vi "Controller Extract FOFB Variables.vi"(8 "error in (no error)":errorcluster, 11 "FOFB Configuration":T1) -> (0 "error out":errorcluster, 3 "FOFB Variables":T10)   [LabVIEW 2011, in "Controller VIs.lvlib"]
uses:
  Controller VIs.lvlib
  Types Definitions/Type FOFB Variables.ctl
  Types Definitions/Type FOFB Configuration.ctl
  Types Definitions/Type FOFB Parameters.ctl
  Types Definitions/Type Network Configuration.ctl
  Types Definitions/Type FA Configuration.ctl
  Types Definitions/Type Response Matrix Measurement Configuration.ctl
  Types Definitions/Type Correction Algorithm Configuration.ctl
  Types Definitions/Type Acquisition Network Configuration.ctl
  Types Definitions/Type Actuation Network Configuration.ctl
  Types Definitions/Type PID Parameters.ctl
  Type Definitions.lvlib
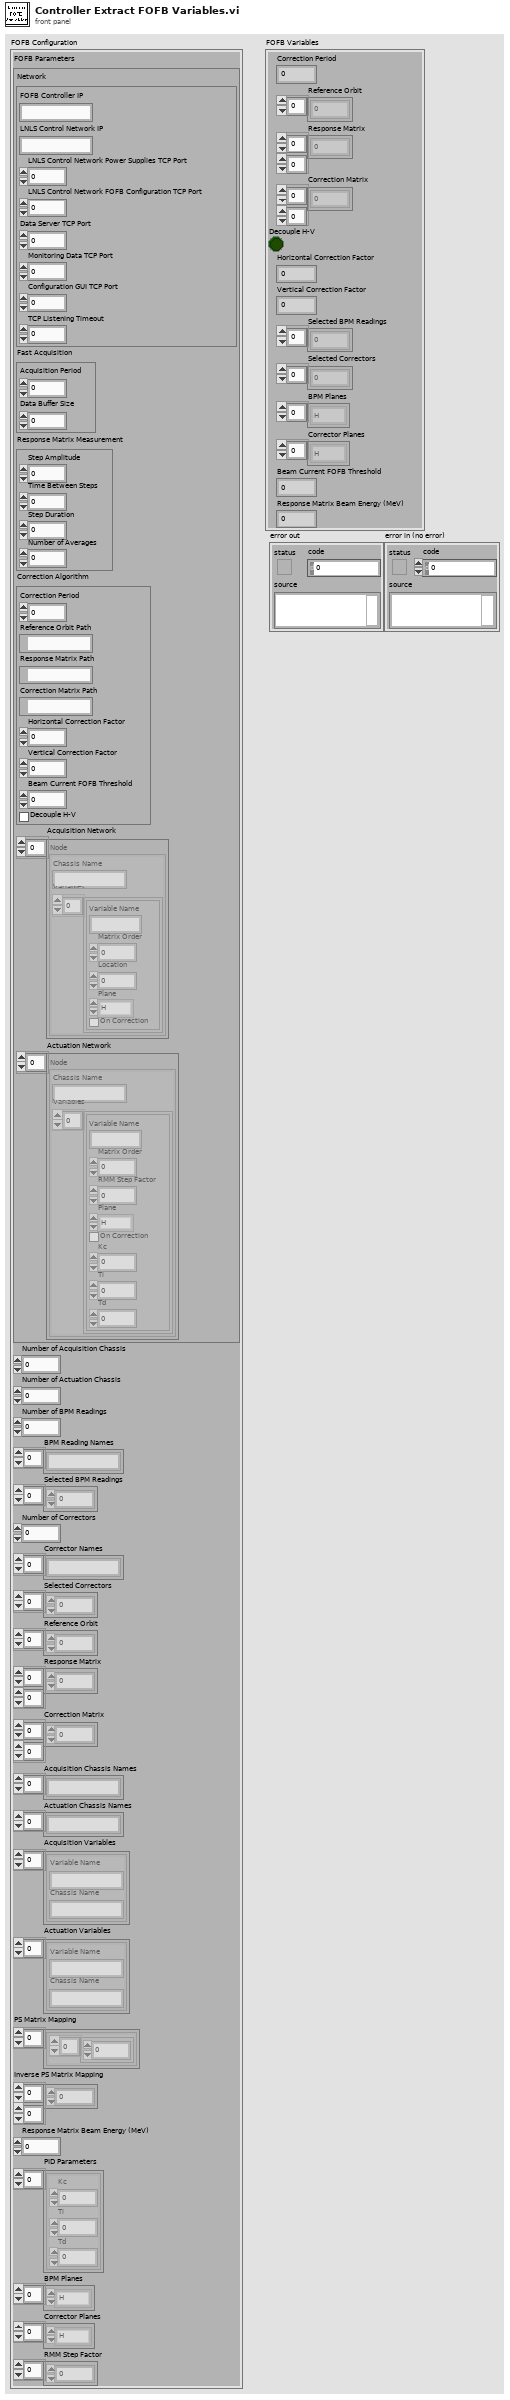
[diagram p1: front panel]
types:
  T1 = typedef "Type Definitions.lvlib/Type FOFB Configuration.ctl" = cluster{"FOFB Parameters":T2, "Number of Acquisition Chassis":i32, "Number of Actuation Chassis":i32, "Number of BPM Readings":i32, "BPM Reading Names":string[], "Selected BPM Readings":u32[], "Number of Correctors":i32, "Corrector Names":string[], "Selected Correctors":u32[], "Reference Orbit":dbl[], "Response Matrix":dbl[][], "Correction Matrix":dbl[][], "Acquisition Chassis Names":string[], "Actuation Chassis Names":string[], "Acquisition Variables":cluster{"Variable Name":string, "Chassis Name":string}[], "Actuation Variables":cluster{"Variable Name":string, "Chassis Name":string}[], "PS Matrix Mapping":cluster{u32[]}[], "Inverse PS Matrix Mapping":u32[][], "Response Matrix Beam Energy (MeV)":dbl, "PID Parameters":T9[], "BPM Planes":enum8{"H", "V"}[], "Corrector Planes":enum8{"H", "V"}[], "RMM Step Factor":dbl[]}
  T2 = typedef "Type Definitions.lvlib/Type FOFB Parameters.ctl" = cluster{"Network":T3, "Fast Acquisition":T4, "Response Matrix Measurement":T5, "Correction Algorithm":T6, "Acquisition Network":T7, "Actuation Network":T8}
  T3 = typedef "Type Definitions.lvlib/Type Network Configuration.ctl" = cluster{"FOFB Controller IP":string, "LNLS Control Network IP":string, "LNLS Control Network Power Supplies TCP Port":u16, "LNLS Control Network FOFB Configuration TCP Port":u16, "Data Server TCP Port":u16, "Monitoring Data TCP Port":u16, "Configuration GUI TCP Port":u16, "TCP Listening Timeout":i32}
  T4 = typedef "Type Definitions.lvlib/Type FA Configuration.ctl" = cluster{"Acquisition Period":u32, "Data Buffer Size":u32}
  T5 = typedef "Type Definitions.lvlib/Type Response Matrix Measurement Configuration.ctl" = cluster{"Step Amplitude":dbl, "Time Between Steps":u32, "Step Duration":u32, "Number of Averages":u32}
  T6 = typedef "Type Definitions.lvlib/Type Correction Algorithm Configuration.ctl" = cluster{"Correction Period":u32, "Reference Orbit Path":path, "Response Matrix Path":path, "Correction Matrix Path":path, "Horizontal Correction Factor":dbl, "Vertical Correction Factor":dbl, "Beam Current FOFB Threshold":dbl, "Decouple H-V":bool}
  T7 = typedef "Type Definitions.lvlib/Type Acquisition Network Configuration.ctl" = cluster{"Chassis Name":string, "Variables":cluster{"Variable Name":string, "Matrix Order":u32, "Location":dbl, "Plane":enum8{"H", "V"}, "On Correction":bool}[]}[]
  T8 = typedef "Type Definitions.lvlib/Type Actuation Network Configuration.ctl" = cluster{"Chassis Name":string, "Variables":cluster{"Variable Name":string, "Matrix Order":u32, "RMM Step Factor":dbl, "Plane":enum8{"H", "V"}, "On Correction":bool, "Kc":dbl, "Ti":dbl, "Td":dbl}[]}[]
  T9 = typedef "Type Definitions.lvlib/Type PID Parameters.ctl" = cluster{"Kc":fxp<+/-,16,8>, "Ti":fxp<+/-,16,8>, "Td":fxp<+/-,16,8>}
  T10 = typedef "Type Definitions.lvlib/Type FOFB Variables.ctl" = cluster{"Correction Period":u32, "Reference Orbit":dbl[], "Response Matrix":dbl[][], "Correction Matrix":dbl[][], "Decouple H-V":bool, "Horizontal Correction Factor":dbl, "Vertical Correction Factor":dbl, "Selected BPM Readings":u32[], "Selected Correctors":u32[], "BPM Planes":enum8{"H", "V"}[], "Corrector Planes":enum8{"H", "V"}[], "Beam Current FOFB Threshold":dbl, "Response Matrix Beam Energy (MeV)":dbl}
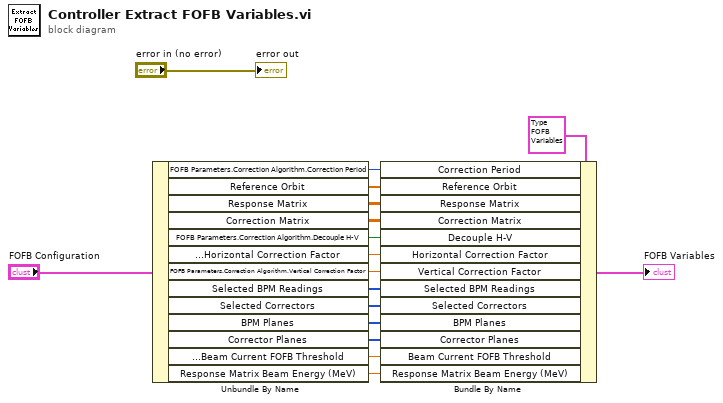
[diagram p0: block diagram]
diagram:
  n1 = Unbundle By Name("FOFB Configuration") -> ("FOFB Parameters.Correction Algorithm.Correction Period"=w15:u32, "Reference Orbit"=w14:dbl[], "Response Matrix"=w13:dbl[][], "Correction Matrix"=w12:dbl[][], "FOFB Parameters.Correction Algorithm.Decouple H-V"=w11:bool, "FOFB Parameters.Correction Algorithm.Horizontal Correction Factor"=w10:dbl, "FOFB Parameters.Correction Algorithm.Vertical Correction Factor"=w9:dbl, "Selected BPM Readings"=w8:u32[], "Selected Correctors"=w7:u32[], "BPM Planes"=w6:enum8{"H", "V"}[], "Corrector Planes"=w5:enum8{"H", "V"}[], "FOFB Parameters.Correction Algorithm.Beam Current FOFB Threshold"=w4:dbl, "Response Matrix Beam Energy (MeV)"=w3:dbl)
  n2 = Bundle By Name(cluster=T10 {"Correction Period"=0, "Reference Orbit"=[], "Response Matrix"=[], "Correction Matrix"=[], "Decouple H-V"=FALSE, "Horizontal Correction Factor"=0.0, "Vertical Correction Factor"=0.0, "Selected BPM Readings"=[], "Selected Correctors"=[], "BPM Planes"=[], "Corrector Planes"=[], "Beam Current FOFB Threshold"=0.0, "Response Matrix Beam Energy (MeV)"=0.0} ("FOFB Variables 2"), "Correction Period"=w15, "Reference Orbit"=w14, "Response Matrix"=w13, "Correction Matrix"=w12, "Decouple H-V"=w11, "Horizontal Correction Factor"=w10, "Vertical Correction Factor"=w9, "Selected BPM Readings"=w8, "Selected Correctors"=w7, "BPM Planes"=w6, "Corrector Planes"=w5, "Beam Current FOFB Threshold"=w4, "Response Matrix Beam Energy (MeV)"=w3) -> (→"FOFB Variables":T10)
  "error out" <- "error in (no error)"
